vi "LoopTime.vi"() -> (3 "LoopTime":u32)   [LabVIEW 2013]
doc: "Measures the time that an external loop requires to execute."
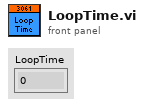
[diagram p1: front panel]
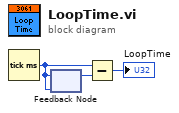
[diagram p0: block diagram]
diagram:
  n1 = Tick Count (ms)() -> (millisecond timer value=w2:u32)
  n2 = feedback-in #1(w2) -> ()
  n3 = feedback #1(w2) -> (w3:u32)
  n4 = Subtract(x=w2, y=w3) -> (x-y=→"LoopTime":u32)
